vi "databasehandle.vi"(7 "condition":string, 8 "error in (no error)":errorcluster caption="错误输入（无错误）", 9 "columns":string[](array[string]), 10 "password":string="123", 11 "table":string) -> (0 "error out":errorcluster caption="错误输出", 3 "data":string[][](array[string]))   [LabVIEW 2016, in "中水三立SQL数据传输.lvlib"]
uses:
  access/access.lvclass
  database_class/database.lvclass/database.ctl
  database_class/database.lvclass
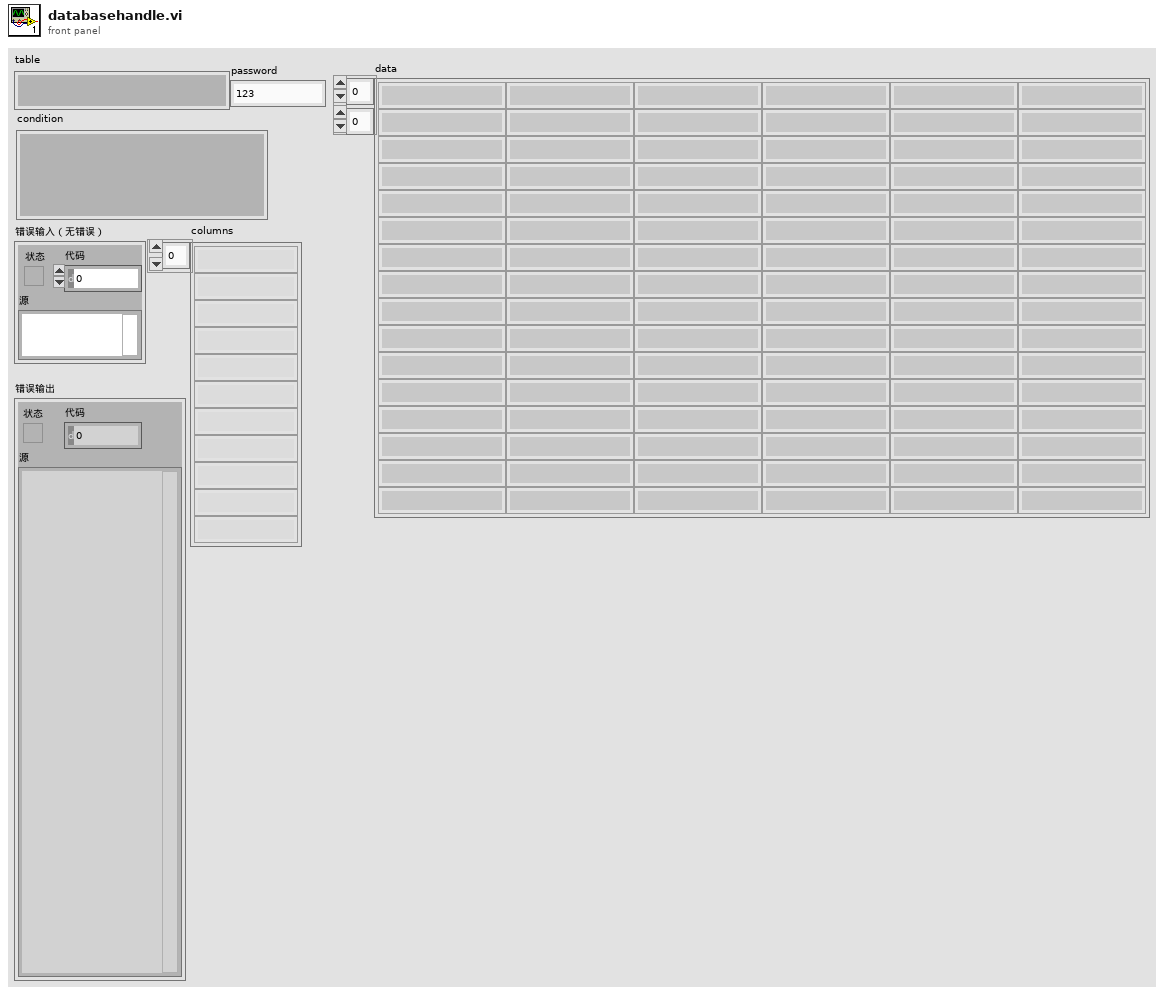
[diagram p1: front panel]
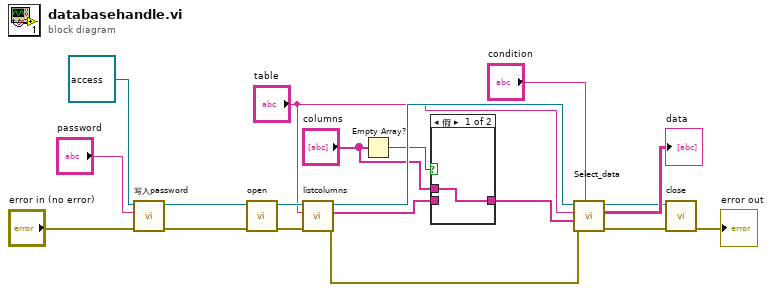
[diagram p0: block diagram]
diagram:
  n1 = call "写入password.vi"("error in (no error)"="error in (no error)", "password"="password", "database输入"=refnum<class "access.lvclass"> refnum ("access.lvclass")) -> ("error out"=w15:errorcluster, "database输出"=w17:refnum<class "access.lvclass">)  [unwired: 7 in]
  n2 = call-dynamic "open.vi"("error in (no error)"=w15, "access 输入"=w17) -> ("error out"=w13:errorcluster, "access 输出"=w14:refnum<class "access.lvclass">)  [unwired: 8 in]
  n3 = call-dynamic "listcolumns.vi"("error in (no error)"=w13, "table"="table", "access 输入"=w14) -> ("error out"=w11:errorcluster, "columns"=w3:string[], "access 输出"=w12:refnum<class "access.lvclass">)  [unwired: 6 in]
  n4 = Empty Array?(array="columns") -> (empty?=w4:bool)
  n5 = case shown="假" w4 {
    tunnel: w3 -> [_ w21]
    tunnel: [w20 w21] -> w2
    tunnel: "columns" -> [w20 _]
    frame False {
    }
    frame True {
    }
  }
  n6 = call-dynamic "Select_data.vi"("condition"="condition", "error in (no error)"=w11, "columns"=w2, "table"="table", "access 输入"=w12) -> ("error out"=w6:errorcluster, "data"=→"data":string[][], "access 输出"=w7:refnum<class "access.lvclass">)  [unwired: 4 in]
  n7 = call-dynamic "close.vi"("error in (no error)"=w6, "access 输入"=w7) -> ("error out"=→"error out":errorcluster)  [unwired: 8 in, 1 out]
